vi "has changed boolen - init first call.vi"(11 "Boolean in":bool) -> (2 "has changed?":bool, 3 "Boolean out":bool)   [LabVIEW 2021, in "RocketPlot.lvlib"]
uses:
  RocketPlot.lvlib
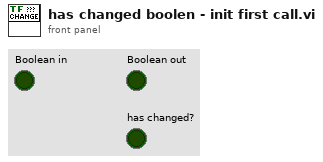
[diagram p1: front panel]
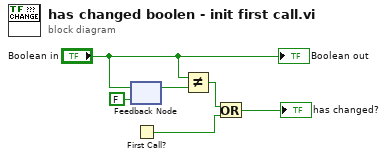
[diagram p0: block diagram]
diagram:
  n1 = feedback-in #1("Boolean in") -> ()
  n2 = feedback #1(FALSE ("Boolean in")) -> (w5:bool)
  n3 = First Call?() -> (First Call?: T/F=w3:bool)
  n4 = Not Equal?(x="Boolean in", y=w5) -> (x != y?=w4:bool)
  n5 = Or(x=w4, y=w3) -> (x .or. y?=→"has changed?":bool)
  "Boolean out" <- "Boolean in"
